vi "Sort Record Entries Debug.vi"(4 "Entries":string[](array[string])) -> (1 "Sorted Entries":string[](array[string]))   [LabVIEW 2013, in "Data Log Fetcher.lvlib"]
uses:
  Data Log Fetcher.lvlib
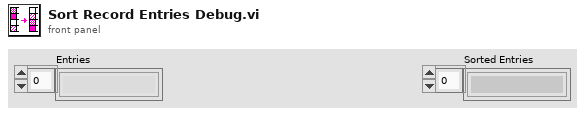
[diagram p1: front panel]
types:
  T1 = enum16{"JAN", "FEB", "MAR", "APR", "MAY", "JUN", "JUL", "AUG", "SEP", "OCT", "NOV", "DEC"}
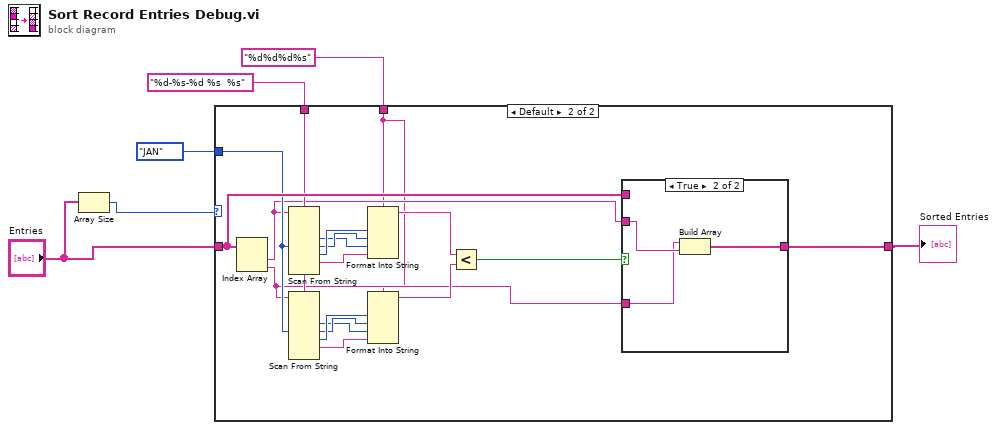
[diagram p0: block diagram]
diagram:
  n1 = Array Size(array="Entries") -> (size(s)=w4:i32)
  n2 = case shown="Default" w4 {
    tunnel: "Entries" -> [w7 w24]
    tunnel: [w7 w25] -> w5
    tunnel: "%d-%s-%d %s  %s" ("format string") -> [_ w23]
    tunnel: T1."JAN" ("Months") -> [_ w22]
    tunnel: "%d%d%d%s" ("format string") -> [_ w8]
    frame 1 {
    }
    frame Default {
      n3 = Index Array(array=w24) -> (element #1=w10:string, element #2=w9:string)  [unwired: 2 in]
      n4 = Scan From String(format string=w23, input string=w10, default 2=w22) -> (output 1=w19:i32, output 2=w20:T1, output 3=w21:i32, output 4=w18:string)  [unwired: 7 in, 3 out]
      n5 = Scan From String(format string=w23, input string=w9, default 2=w22) -> (output 1=w15:i32, output 2=w16:T1, output 3=w17:i32, output 4=w14:string)  [unwired: 7 in, 3 out]
      n6 = Format Into String(format string=w8, w21, w20, w19, w18) -> (resulting string=w13:string)  [unwired: 2 in, 1 out]
      n7 = Format Into String(format string=w8, w17, w16, w15, w14) -> (resulting string=w12:string)  [unwired: 2 in, 1 out]
      n8 = Less?(x=w13, y=w12) -> (x < y?=w11:bool)
      n9 = case shown="True" w11 {
        tunnel: [w26 w29] -> w25
        tunnel: w10 -> [_ w28]
        tunnel: w9 -> [_ w27]
        tunnel: w24 -> [w26 _]
        frame False {
        }
        frame True {
          n10 = Build Array(w27, w28) -> (w29:string[])
        }
      }
    }
  }
  "Sorted Entries" <- w5
